vi "InitPneumatics.vi"   [LabVIEW 2019]
doc: "This VI initializes subsytem-agnostic pneumatic devices."
uses:
  <vilib>/Rock Robotics/WPI/Utilities/WPI_GetSetVariantRefNum.vi
  refnums.vi
types:
  T1 = typedef "WPI_CompressorDevRef.ctl" = cluster{"DevStatus":errorcluster, "Pneumatics Control Module":u8}
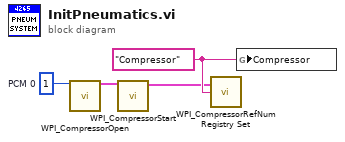
[diagram p0: block diagram]
diagram:
  w4 = "Compressor" ("refnum name")
  w2 = u8 1  # PCM 0
  n1 = call <vilib>:"WPI_CompressorOpen.vi"("Pneumatics Control Module (0)"=w2) -> ("CompressorDevRef"=w1:T1)  [unwired: 13 in, 1 out]
  n2 = call <vilib>:"WPI_CompressorStart.vi"("CompressorDevRef"=w1) -> ("CompressorDevRef"=w3:T1)  [unwired: 9 in, 1 out]
  n3 = call <vilib>:"WPI_CompressorRefNum Registry Set.vi"("refnum name"=w4, "CompressorDevRef"=w3) -> ()  [unwired: 8 in, 2 out]
  n4 = global write "refnums.vi" "Compressor"(w4) -> ()
